vi "HB_DisplayLCD.vi"(4 "LCD Backlight":T1(ring), 6 "Clear LCD Display":bool=TRUE, 8 "error in (no error)":errorcluster, 10 "Display String":string, 11 "HBDeviceRef":T2) -> (0 "error out":errorcluster, 3 "HBDeviceRef":T2)   [LabVIEW 2016]
doc: "Displays the specified string on the configured LCD. The LCD must be connected to the HB LCD channel on the Huskie Board. By default, the LCD display is cleared before the string is written. An optional control allows the backlight of the LCD to be enabled, disabled, or left unchanged.\n\nFor more advanced operations with the Parallax LCDs, the following control codes are supported:\n LCD_RT = $09 ' move cursor right\n LCD_LF = $0A ' move cursor down 1 line\n LCD_CLS = $0C ' clear LCD (follow with 5 ms delay)\n LCD_CR = $0D ' move pos 0 of next line\n LCD_BL_ON = $11 ' backlight on\n LCD_BL_OFF = $12 ' backlight off\n LCD_OFF = $15 ' LCD off\n LCD_ON1 = $16 ' LCD on; cursor off, blink off\n LCD_ON2 = $17 ' LCD on; cursor off, blink on\n LCD_ON3 = $18 ' LCD on; cursor on, blink off\n LCD_ON4 = $19 ' LCD on; cursor on, blink on"
uses:
  <vilib>/Rock Robotics/WPI/SerialPort/WPI_SerialPortRef.ctl
  <vilib>/Utility/error.llb/Error Cluster From Error Code.vi
  <vilib>/ErrorRing/Error Ring.xnode
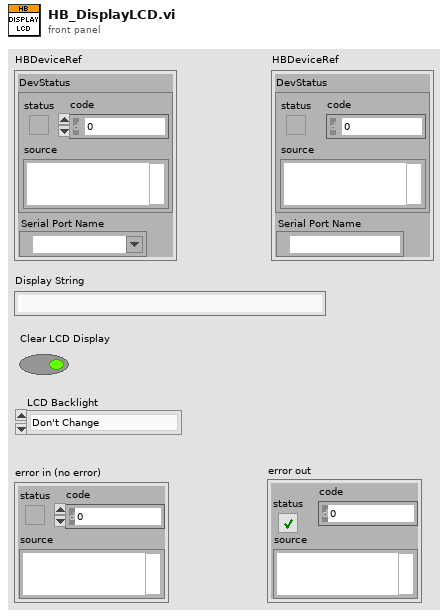
[diagram p1: front panel]
types:
  T1 = enum8{"Don't Change", "Backlight On", "Backlight Off"}
  T2 = typedef "WPI_SerialPortRef.ctl" = cluster{"DevStatus":errorcluster, "Serial Port Name":refnum<visa-resource-name>}
  T3 = enum16{"Native", "Native Command Line", "UNIX", "Macintosh", "DOS"}
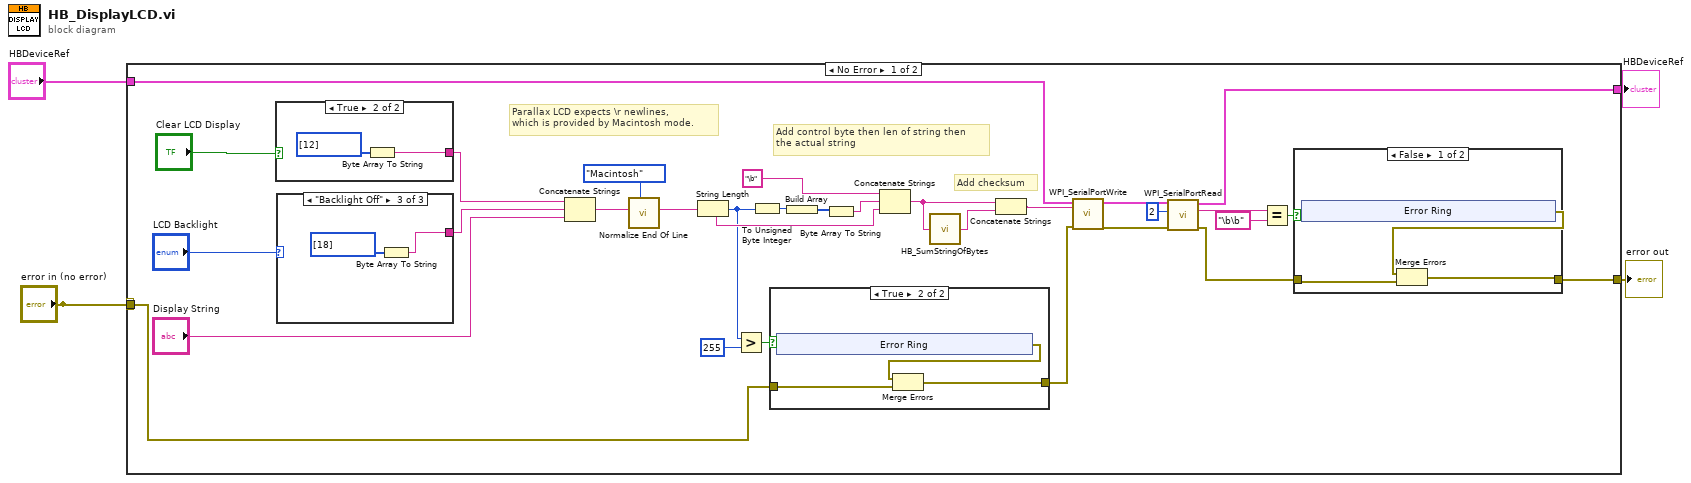
[diagram p0: block diagram]
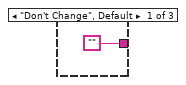
[diagram p3: hidden frame]
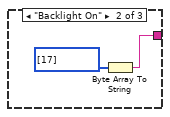
[diagram p4: hidden frame]
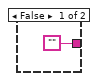
[diagram p5: hidden frame]
diagram:
  n1 = case shown="No Error" "error in (no error)" {
    selector: "error in (no error)" -> [_ w60]
    tunnel: "HBDeviceRef" -> [w34 w59]
    tunnel: "error in (no error)" -> [w6 _]
    tunnel: [w31 w59] -> w3
    tunnel: [w25 w60] -> w2
    frame No Error {
      # "Parallax LCD expects \\r newlines, \nwhich is provided by Macintosh mode."
      # "Add checksum"
      # "Add control byte then len of string then \nthe actual string"
      n2 = case shown="True" "Clear LCD Display" {
        tunnel: ["" w49] -> w12
        frame False {
        }
        frame True {
          n3 = Byte Array To String(unsigned byte array=u8[] [12]) -> (string=w49:string)
        }
      }
      n4 = case shown="\"Backlight Off\"" "LCD Backlight" {
        tunnel: ["" w44 w46] -> w11
        frame "Don't Change", Default {
        }
        frame "Backlight On" {
          n5 = Byte Array To String(unsigned byte array=u8[] [17]) -> (string=w44:string)
        }
        frame "Backlight Off" {
          n6 = Byte Array To String(unsigned byte array=u8[] [18]) -> (string=w46:string)
        }
      }
      n7 = Concatenate Strings(w12, w11, "Display String") -> (w13:string)
      n8 = call <vilib>:"Normalize End Of Line.vi"("end of line (Native)"=T3."Macintosh", "string in"=w13) -> ("string out"=w16:string)  [unwired: 6 in]
      n9 = String Length(string=w16) -> (length=w8:i32)
      n10 = Greater?(x=w8, y=255) -> (0:w9:bool)
      n11 = To Unsigned Byte Integer(number=w8) -> (unsigned 8bit integer=w22:u8)
      n12 = case shown="True" w9 {
        tunnel: w6 -> [w35 w37]
        tunnel: [w35 w36] -> w5
        frame False {
        }
        frame True {
          n13 = xnode "Error Ring"() -> ("error out"=w38:errorcluster)
          n14 = Merge Errors(w38, w37) -> (w36:errorcluster)
        }
      }
      n15 = Build Array(w22) -> (w23:u8[])
      n16 = Byte Array To String(unsigned byte array=w23) -> (string=w24:string)
      n17 = Concatenate Strings("\b", w24, w16) -> (w19:string)
      n18 = call "HB_SumStringOfBytes.vi"("String Of Bytes"=w19) -> ("Sum as String"=w18:string)
      n19 = Concatenate Strings(w19, w18) -> (w20:string)
      n20 = call <vilib>:"WPI_SerialPortWrite.vi"("error in (no error)"=w5, "Buffer"=w20, "SerialPortRef"=w34) -> ("error out"=w32:errorcluster, "SerialPortRef"=w33:T2)  [unwired: 6 in, 1 out]
      n21 = call <vilib>:"WPI_SerialPortRead.vi"("error in (no error)"=w32, "Num Bytes to Read"=u32 2, "SerialPortRef"=w33) -> ("error out"=w26:errorcluster, "Buffer"=w29:string, "SerialPortRef"=w31:T2)  [unwired: 6 in]
      n22 = Equal?(x=w29, y="\b\b") -> (x = y?=w27:bool)
      n23 = case shown="False" w27 {
        tunnel: w26 -> [w52 w58]
        tunnel: [w53 w58] -> w25
        frame False {
          n24 = xnode "Error Ring"() -> ("error out"=w51:errorcluster)
          n25 = Merge Errors(w51, w52) -> (w53:errorcluster)
        }
        frame True {
        }
      }
    }
    frame Error {
    }
  }
  "HBDeviceRef" <- w3
  "error out" <- w2
